vi "get_enum.vi"(11 "path":string) -> (0 "error out":errorcluster, 3 "Enum Elements":string[](array[string]))   [LabVIEW 2026, in "G-AI Core.lvlib"]
doc: "Returns the elements of an enum stored in a .ctl file specified by path. Use this to see which elements a type-defined enum has."
uses:
  G-AI Core.lvlib
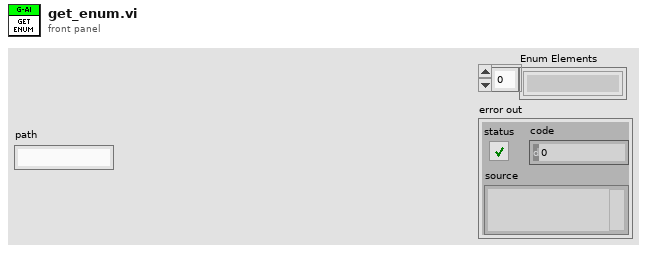
[diagram p1: front panel]
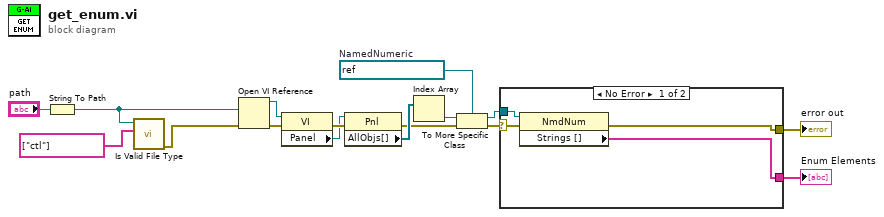
[diagram p0: block diagram]
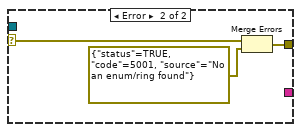
[diagram p2: hidden frame]
diagram:
  w7 = refnum<vi> refnum  # NamedNumeric
  n1 = String To Path(string="path") -> (path=w3:path)
  n2 = call "Is Valid File Type.vi"("y"=string[] ["ctl"], "Path"=w3) -> ("error out"=w2:errorcluster)  [unwired: 9 in]
  n3 = Open VI Reference(vi path=w3, error in (no error)=w2) -> (vi reference=w14:refnum<vi>, error out=w15:errorcluster)  [unwired: 4 in]
  n4 = property class="VI"(reference=w14, error in=w15) -> (error out=w13:errorcluster, "Panel"=w12:refnum<vi>)  [unwired: 1 out]
  n5 = property class="Pnl"(reference=w12, error in=w13) -> (error out=w10:errorcluster, "AllObjs[]"=w11:refnum<vi>[])  [unwired: 1 out]
  n6 = Index Array(array=w11) -> (element=w9:refnum<vi>)  [unwired: 1 in]
  n7 = To More Specific Class(target class=w7, reference=w9, error in=w10) -> (specific class reference=w8:refnum<vi>, error out=w4:errorcluster)
  n8 = case shown="No Error" w4 {
    selector: w4 -> [w17 w21]
    tunnel: w8 -> [w20 _]
    tunnel: [w19 _] -> w6
    tunnel: [w18 w22] -> w5
    frame No Error {
      n9 = property class="NmdNum"(reference=w20, error in=w17) -> (error out=w18:errorcluster, "Strings []"=w19:string[])  [unwired: 1 out]
    }
    frame Error {
      n10 = Merge Errors(w21, errorcluster {"status"=TRUE, "code"=5001, "source"="No an enum/ring found"} ("error out")) -> (w22:errorcluster)
    }
  }
  "Enum Elements" <- w6
  "error out" <- w5
